vi "Keys.vi"(8 "error in (no error)":errorcluster, 11 "Array In":refnum<class "Array.lvclass">) -> (0 "error out":errorcluster, 2 "Keys":string[](array[string]), 3 "Array Out":refnum<class "Array.lvclass">)   [LabVIEW 2013, in "LapDog.Collections.v1.Maps.Implementations.lvlib" / "Array.lvclass"]
doc: "Returns a copy of all keys in the map."
uses:
  Array.lvclass
  Array.lvclass/Array.ctl
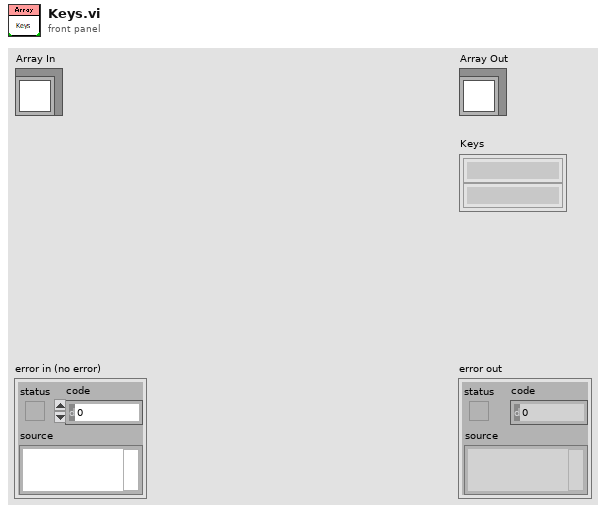
[diagram p1: front panel]
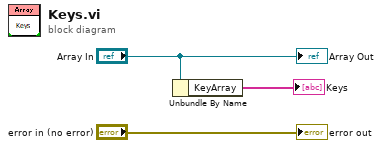
[diagram p0: block diagram]
diagram:
  n1 = Unbundle By Name("Array In") -> ("KeyArray"=→"Keys":string[])
  "error out" <- "error in (no error)"
  "Array Out" <- "Array In"
